vi "TDT-Load and Run Circuit.vi"(0 "RPcox In":refnum<k7>, 5 "Circuit File":string, 9 "SampFreq":dbl format="%#_9g", 11 "error in (no error)":errorcluster) -> (4 "RPcox Out":refnum<k7>, 15 "error out":errorcluster)   [LabVIEW 2015]
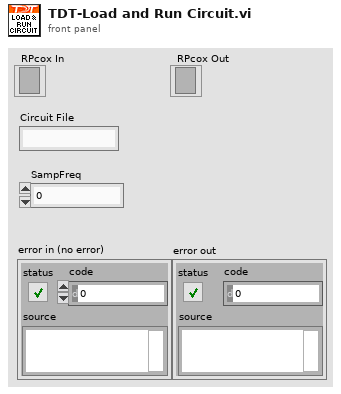
[diagram p1: front panel]
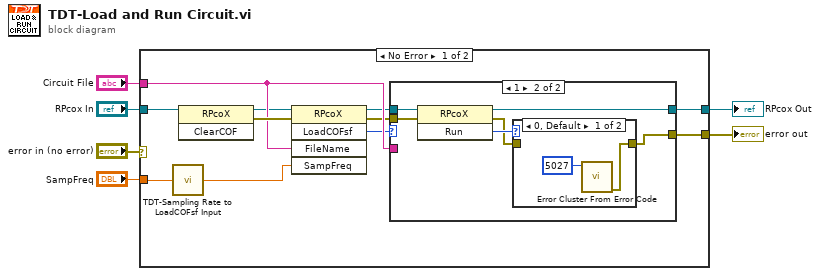
[diagram p0: block diagram]
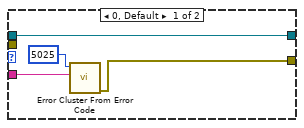
[diagram p2: hidden frame]
diagram:
  n1 = case shown="No Error" "error in (no error)" {
    selector: "error in (no error)" -> [_ w31]
    tunnel: "Circuit File" -> [w16 _]
    tunnel: [w11 w31] -> w5
    tunnel: [w10 w32] -> w4
    tunnel: "RPcox In" -> [w9 w32]
    tunnel: "SampFreq" -> [w8 _]
    frame No Error {
      n2 = call "TDT-Sampling Rate to LoadCOFsf Input.vi"("Sampling rate (Hz)"=w8) -> ("LoadCOFsf Input"=w7:dbl)  [unwired: 14 in]
      n3 = invoke class="RPcoX" method="ClearCOF"(reference=w9) -> (reference out=w15:refnum<k7>, error out=w17:errorcluster)  [unwired: 2 in, 1 out]
      n4 = invoke class="RPcoX" method="LoadCOFsf"(reference=w15, error in=w17, "FileName"=w16, "SampFreq"=w7) -> (reference out=w13:refnum<k7>, error out=w14:errorcluster, "LoadCOFsf"=w12:i32)  [unwired: 1 in, 2 out]
      n5 = case shown="1" w12 {
        tunnel: w16 -> [w20 _]
        tunnel: w13 -> [w21 w27]
        tunnel: w14 -> [_ w26]
        tunnel: [w21 w25] -> w10
        tunnel: [w18 w22] -> w11
        frame 0, Default {
          n6 = call <vilib>:"Error Cluster From Error Code.vi"("error message (\"\")"=w20, "error code (0)"=5025) -> ("error out"=w18:errorcluster)  [unwired: 7 in]
        }
        frame 1 {
          n7 = invoke class="RPcoX" method="Run"(reference=w27, error in=w26) -> (reference out=w25:refnum<k7>, error out=w23:errorcluster, "Run"=w24:i32)  [unwired: 1 in]
          n8 = case shown="0, Default" w24 {
            tunnel: [w28 w30] -> w22
            tunnel: w23 -> [_ w30]
            frame 0, Default {
              n9 = call <vilib>:"Error Cluster From Error Code.vi"("error code (0)"=5027) -> ("error out"=w28:errorcluster)  [unwired: 8 in]
            }
            frame 1 {
            }
          }
        }
      }
    }
    frame Error {
    }
  }
  "error out" <- w5
  "RPcox Out" <- w4
